vi "Handle Error.vi"(8 "error in (no error)":errorcluster, 11 "Assert Display in":refnum<class "Assert Display.lvclass">) -> (0 "error out":errorcluster, 2 "stop actor?":bool=TRUE, 3 "Assert Display out":refnum<class "Assert Display.lvclass">)   [LabVIEW 2016, in "Assert API Components.lvlib" / "Assert Display.lvlib" / "Assert Display.lvclass"]
doc: "(<B>Filename</B>: Actor Framework.lvlib:Actor.lvclass:Handle Error.vi)\n\nDefines how the actor handles an error that occurred while processing a message. By default, this method does nothing except stop the actor."
uses:
  Assert Display.lvclass
  Base UI Actor/Base UI Actor/Base UI Actor.lvclass
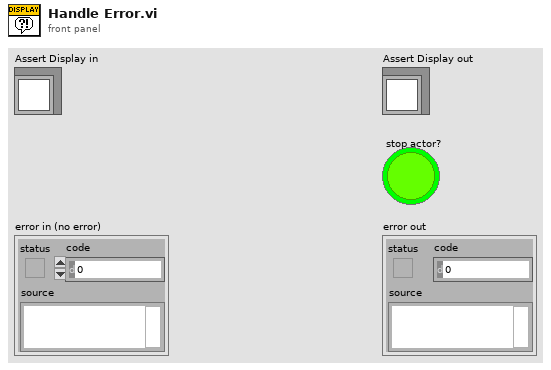
[diagram p1: front panel]
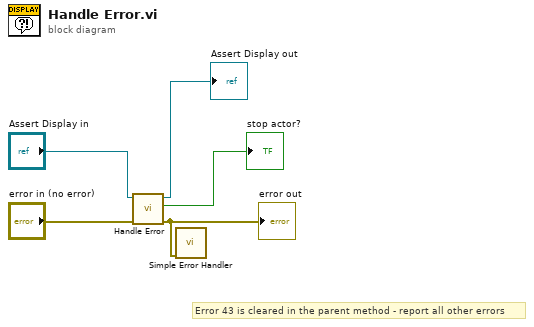
[diagram p0: block diagram]
diagram:
  # "Error 43 is cleared in the parent method - report all other errors"
  n1 = call-parent "Handle Error.vi"("error in (no error)"="error in (no error)", "Actor in"="Assert Display in") -> ("error out"=w1:errorcluster, "stop actor?"=→"stop actor?":bool, "Actor out"=→"Assert Display out":refnum<class "Assert Display.lvclass">)  [unwired: 7 in]
  "error out" <- w1
  n2 = call <vilib>:"Simple Error Handler.vi"("error in (no error)"=w1) -> ()  [unwired: 4 in, 5 out]
